vi "9_GuessingGame.vi"() -> ()   [LabVIEW 2015]
panel:
  out "message":string
  out "Number of guesses so far":i32
  out "Correct!":bool
  in  "OK Button":bool
  in  "Number to guess (1-100)":i32
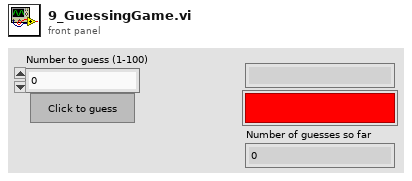
[diagram p1: front panel]
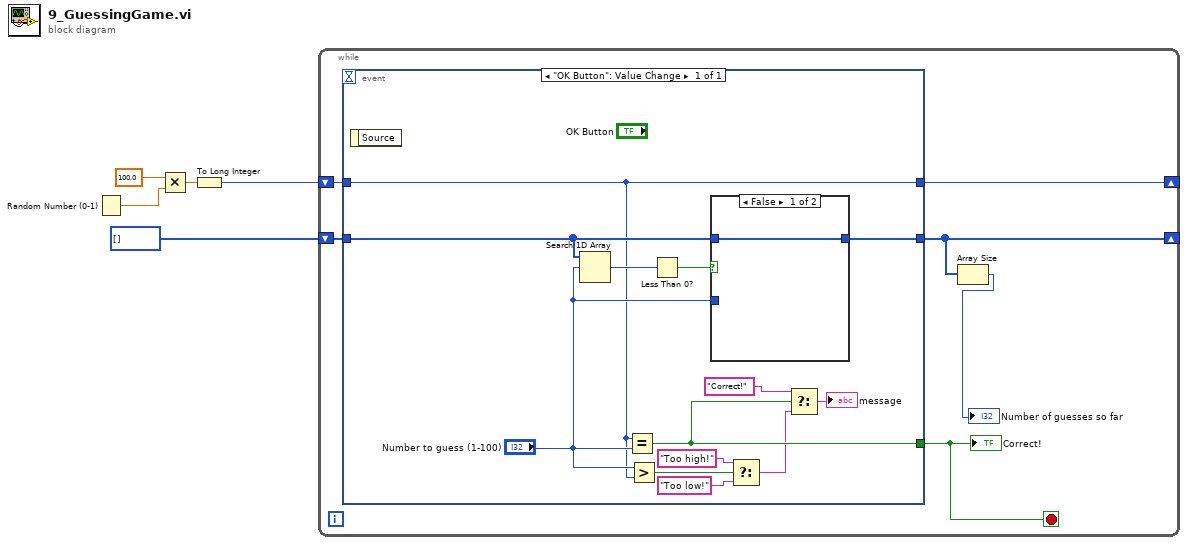
[diagram p0: block diagram]
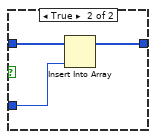
[diagram p2: hidden frame]
diagram:
  n1 = Random Number (0-1)() -> (number: 0 to 1=w4:dbl)
  n2 = Multiply(x=100.0, y=w4) -> (x*y=w3:dbl)
  n3 = To Long Integer(number=w3) -> (32bit integer=w2:i32)
  n4 = while {
    shift-right: [w8] -> _
    shift-left: w2 -> [w10]
    shift-right: [w7] -> _
    shift-left: i32[] [] -> [w9]
    stop <- w11 stop-if-true
    n5 = event shown="[0] \"OK Button\": Value Change" {
      selector: _ -> [_]
      dyn-events: _ -> [_]
      timeout: _ -> [_]
      tunnel: [w24] -> w11
      tunnel: w10 -> [w16]
      tunnel: w9 -> [w19]
      tunnel: [w16] -> w8
      tunnel: [w18] -> w7
      event "OK Button": Value Change {
        n6 = event-data() -> ()  [unwired: 1 in, 1 out]
        n7 = Search 1D Array(1D array=w19, element="Number to guess (1-100)") -> (index of element=w21:i32)  [unwired: 1 in]
        n8 = Equal?(x=w16, y="Number to guess (1-100)") -> (x = y?=w24:bool)
        n9 = Greater?(x="Number to guess (1-100)", y=w16) -> (0:w15:bool)
        n10 = Less Than 0?(x=w21) -> (x < 0?=w20:bool)
        n11 = case shown="False" w20 {
          tunnel: w19 -> [w25 w28]
          tunnel: "Number to guess (1-100)" -> [_ w27]
          tunnel: [w25 w26] -> w18
          frame False {
          }
          frame True {
            n12 = Insert Into Array(array=w28, new element=w27) -> (w26:i32[])  [unwired: 1 in]
          }
        }
        n13 = Select(t="Too high!", s=w15, f="Too low!") -> (s? t:f=w12:string)
        n14 = Select(t="Correct!", s=w24, f=w12) -> (s? t:f=→"message":string)
      }
    }
    "Correct!" <- w11
    n15 = Array Size(array=w7) -> (size(s)=→"Number of guesses so far":i32)
  }
